vi "UTF8ToASCII.vi"(8 "错误输入":errorcluster, 11 "utf-8文本":string) -> (0 "错误输出":errorcluster, 3 "文本":string)   [LabVIEW 2020, in "Other.lvlib"]
uses:
  Other.lvlib
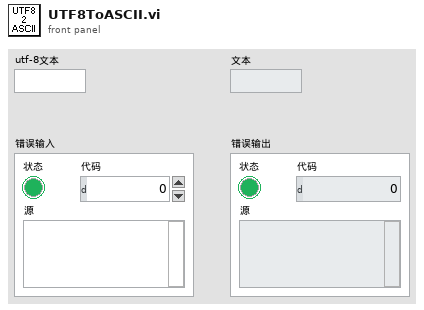
[diagram p1: front panel]
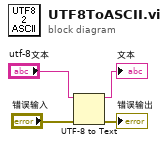
[diagram p0: block diagram]
diagram:
  n1 = UTF-8 to Text(8:"错误输入", 11:"utf-8文本") -> (0:→"错误输出":errorcluster, 3:→"文本":string)  [unwired: 1 in]
